vi "RB_Risize.vi"(2 "error in (no error)":errorcluster caption="错误输入（无错误）", 3 "本VI":refnum<vi>) -> (0 "error out":errorcluster caption="错误输出")   [LabVIEW 2012]
uses:
  <vilib>/Utility/inputDevices.llb/mouseAcquire.vi
  <vilib>/Utility/inputDevices.llb/closeMouse.vi
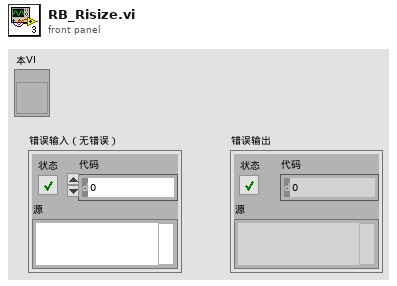
[diagram p1: front panel]
types:
  T1 = cluster{"Horizontal":i32, "Vertical":i32, "Scrolling":i32}
  T2 = cluster{"button 1":bool, "button 2":bool, "button 3":bool, "button 4":bool}
  T3 = typedef "LVRectTypeDef.ctl" = cluster{"Left":i16, "Top":i16, "Right":i16, "Bottom":i16}
  T4 = cluster{"Left":i16, "Top":i16, "Horizontal":i32, "Vertical":i32}
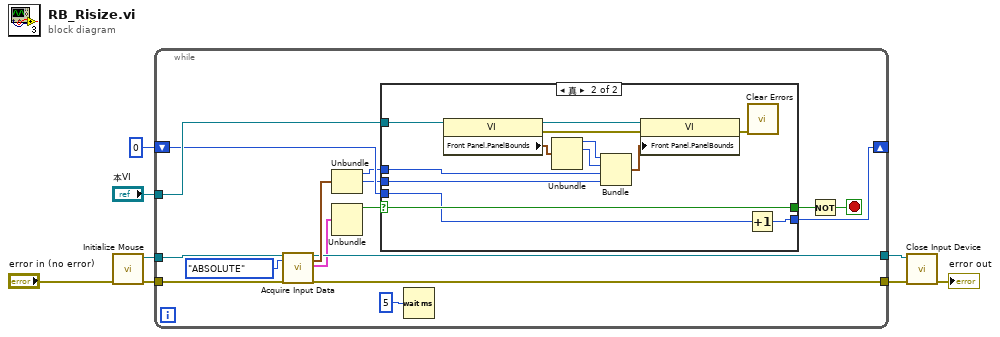
[diagram p0: block diagram]
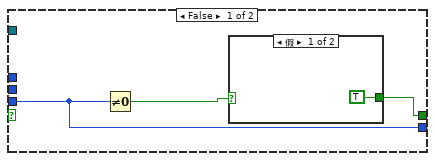
[diagram p2: hidden frame]
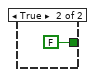
[diagram p3: hidden frame]
diagram:
  n1 = call <vilib>:"Initialize Mouse.vi"("error in (no error)"="error in (no error)") -> ("error out"=w7:errorcluster, "device ID"=w8:refnum<k1>)  [unwired: 9 in]
  n2 = while {
    tunnel: w8 -> [w23]
    tunnel: w7 -> [w22]
    tunnel: [w20] -> w6
    tunnel: [w19] -> w5
    tunnel: "本VI" -> [w15]
    shift-right: [w11] -> _
    shift-left: u32 0 ("等待时间（毫秒）") -> [w12]
    stop <- w13 stop-if-true
    n3 = call-poly <vilib>:"Acquire Input Data.vi"("device ID"=w23, "key mode"=enum16{"RELATIVE", "ABSOLUTE"}."ABSOLUTE", "error in (no error)"=w22) -> ("device ID"=w20:refnum<k1>, "axis info"=w21:T1, "button info"=w18:T2, "error out"=w19:errorcluster)  [unwired: 13 in]
    n4 = Unbundle(w21) -> ("Horizontal"=w10:i32, "Vertical"=w9:i32)  [unwired: 1 out]
    n5 = Unbundle(w18) -> ("button 1"=w17:bool)  [unwired: 3 out]
    n6 = case shown="真" w17 {
      selector: w17 -> [_ w38]
      tunnel: w10 -> [_ w31]
      tunnel: w15 -> [_ w39]
      tunnel: [w27 w38] -> w14
      tunnel: w12 -> [w25 w37]
      tunnel: [w25 w36] -> w11
      tunnel: w9 -> [_ w30]
      frame False {
        n7 = Not Equal To 0?(x=w25) -> (x != 0?=w26:bool)
        n8 = case shown="假" w26 {
          tunnel: [TRUE FALSE] -> w27
          frame False {
          }
          frame True {
          }
        }
      }
      frame True {
        n9 = property class="VI"(reference=w39) -> (reference out=w42:refnum<vi>, error out=w35:errorcluster, "Front Panel.PanelBounds"=w41:T3)  [unwired: 1 in]
        n10 = Unbundle(w41) -> ("Left"=w33:i16, "Top"=w32:i16)  [unwired: 2 out]
        n11 = Bundle("Left"=w33, "Top"=w32, "Horizontal"=w31, "Vertical"=w30) -> (w40:T4)  [unwired: 1 in]
        n12 = property class="VI"(reference=w42, error in=w35, "Front Panel.PanelBounds"=w40) -> (error out=w34:errorcluster)  [unwired: 1 out]
        n13 = Increment(x=w37) -> (x+1=w36:u32)
        n14 = call <vilib>:"Clear Errors.vi"("error in (no error)"=w34) -> ()  [unwired: 6 in, 1 out]
      }
    }
    n15 = Wait (ms)(milliseconds to wait=u32 5 ("等待时间（毫秒）")) -> ()  [unwired: 1 out]
    n16 = Not(x=w14) -> (.not. x?=w13:bool)
  }
  n17 = call-poly <vilib>:"Close Input Device.vi"("error in (no error)"=w5, "device ID"=w6) -> ("error out"=→"error out":errorcluster)  [unwired: 8 in]
